vi "emi_BW 8Bit image to Linear DuoTone.vi"(0 "BW Image in":T1, 5 "Dark(Black)":u32(colorbox), 7 "Light(White)":u32(colorbox)=16448250, 11 "error in (no error)":errorcluster) -> (4 "Duotone Image out":T1, 15 "error out":errorcluster)   [LabVIEW 2011]
doc: "Acceps a BW 8 bit image, and two colors. It creates a duo tone image based on these. \n\nIntended use: Color gradiants.s\n\nOn Error: No action"
uses:
  <vilib>/picture/picture.llb/imagedata.ctl
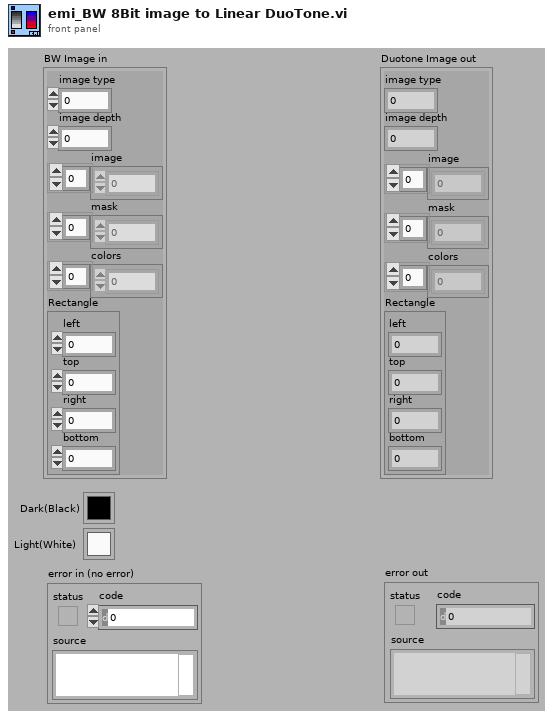
[diagram p1: front panel]
types:
  T1 = typedef "imagedata.ctl" = cluster{"image type":i32, "image depth":i32, "image":u8[], "mask":u8[], "colors":u32[], "Rectangle":cluster{"left":i16, "top":i16, "right":i16, "bottom":i16}}
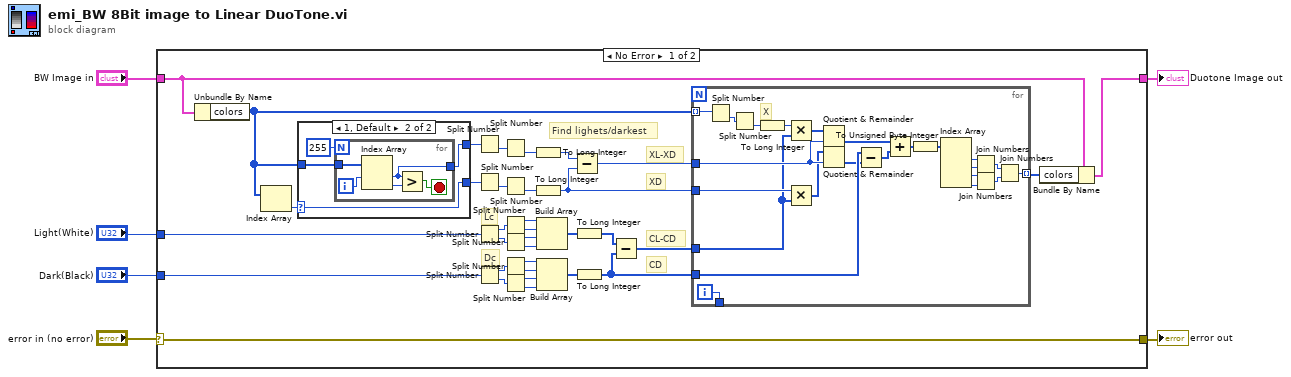
[diagram p0: block diagram]
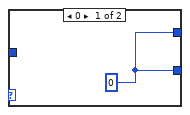
[diagram p2: hidden frame]
diagram:
  n1 = case shown="No Error" "error in (no error)" {
    selector: "error in (no error)" -> [w7 w75]
    tunnel: [w40 w74] -> w6
    tunnel: "BW Image in" -> [w39 w74]
    tunnel: "Light(White)" -> [w38 _]
    tunnel: "Dark(Black)" -> [w37 _]
    tunnel: [w7 w75] -> w1
    frame No Error {
      # "Find lighets/darkest"
      # "CD"
      # "XD"
      # "XL-XD"
      # "CL-CD"
      # "Dc"
      # "Lc"
      n2 = Unbundle By Name(w39) -> ("colors"=w33:u32[])
      n3 = Index Array(array=w33) -> (element=w34:u32)  [unwired: 1 in]
      n4 = case shown="1, Default" w34 {
        selector: w34 -> [_ w42]
        tunnel: w33 -> [_ w43]
        tunnel: [w41 w44] -> w35
        tunnel: [w41 w42] -> w36
        frame 0 {
          w41 = u32 0
          # "Colors starter med 0, mao bare en farge, sort"
        }
        frame 1, Default {
          n5 = for {
            N: 255 -> [_]
            tunnel: w43 -> [w49]
            tunnel: [w46] -> w44
            i -> [w50]
            stop <- w47 stop-if-true
            n6 = Index Array(array=w49, index #1=w50) -> (element #1=w46:u32, element #2=w48:u32)  [unwired: 1 in]
            n7 = Greater?(x=w46, y=w48) -> (0:w47:bool)
          }
        }
      }
      n8 = Split Number(x=w35) -> (lo(x)=w20:u16)  [unwired: 1 out]
      n9 = Split Number(x=w36) -> (lo(x)=w21:u16)  [unwired: 1 out]
      n10 = Split Number(x=w38) -> (hi(x)=w19:u16, lo(x)=w18:u16)
      n11 = Split Number(x=w37) -> (hi(x)=w8:u16, lo(x)=w9:u16)
      n12 = Split Number(x=w20) -> (lo(x)=w22:u8)  [unwired: 1 out]
      n13 = Split Number(x=w21) -> (lo(x)=w29:u8)  [unwired: 1 out]
      n14 = Split Number(x=w19) -> (hi(x)=w17:u8, lo(x)=w16:u8)
      n15 = Split Number(x=w18) -> (hi(x)=w15:u8, lo(x)=w14:u8)
      n16 = Split Number(x=w8) -> (hi(x)=w10:u8, lo(x)=w11:u8)
      n17 = Split Number(x=w9) -> (hi(x)=w12:u8, lo(x)=w13:u8)
      n18 = To Long Integer(number=w22) -> (32bit integer=w30:i32)
      n19 = To Long Integer(number=w29) -> (32bit integer=w31:i32)
      n20 = Build Array(w17, w16, w15, w14) -> (w23:u8[])
      n21 = Build Array(w10, w11, w12, w13) -> (w24:u8[])
      n22 = Subtract(x=w30, y=w31) -> (x-y=w28:i32)
      n23 = To Long Integer(number=w23) -> (32bit integer=w26:i32[])
      n24 = To Long Integer(number=w24) -> (32bit integer=w27:i32[])
      n25 = Subtract(x=w26, y=w27) -> (x-y=w25:i32[])
      n26 = for {
        tunnel: w33 -> [w73] mode=indexing
        tunnel: [w71] -> w32 mode=indexing
        tunnel: [w72] -> _
        tunnel: w27 -> [w69]
        tunnel: w31 -> [w70]
        tunnel: w28 -> [w68]
        tunnel: w25 -> [w67]
        i -> [w72]
        # "X"
        n27 = Split Number(x=w73) -> (lo(x)=w66:u16)  [unwired: 1 out]
        n28 = Split Number(x=w66) -> (lo(x)=w53:u8)  [unwired: 1 out]
        n29 = To Long Integer(number=w53) -> (32bit integer=w55:i32)
        n30 = Multiply(x=w55, y=w67) -> (x*y=w56:i32[])
        n31 = Multiply(x=w70, y=w67) -> (x*y=w54:i32[])
        n32 = Quotient & Remainder(x=w56, y=w68) -> (floor(x/y)=w57:i32[])  [unwired: 1 out]
        n33 = Quotient & Remainder(x=w54, y=w68) -> (floor(x/y)=w52:i32[])  [unwired: 1 out]
        n34 = Subtract(x=w69, y=w52) -> (x-y=w65:i32[])
        n35 = Add(x=w57, y=w65) -> (x+y=w58:i32[])
        n36 = To Unsigned Byte Integer(number=w58) -> (unsigned 8bit integer=w51:u8[])
        n37 = Index Array(array=w51) -> (element #1=w60:u8, element #2=w64:u8, element #3=w63:u8, element #4=w59:u8)  [unwired: 4 in]
        n38 = Join Numbers(hi=w60, lo=w64) -> ((hi.lo)=w61:u16)
        n39 = Join Numbers(hi=w63, lo=w59) -> ((hi.lo)=w62:u16)
        n40 = Join Numbers(hi=w61, lo=w62) -> ((hi.lo)=w71:u32)
      }
      n41 = Bundle By Name(cluster=w39, "colors"=w32) -> (w40:T1)
    }
    frame Error {
    }
  }
  "Duotone Image out" <- w6
  "error out" <- w1
